vi "Read Error Logger's Enqueuer.vi"(8 "error in (no error)":errorcluster, 11 "TCP_Listener in":refnum<class "TCP_Listener.lvclass">) -> (0 "error out":errorcluster, 2 "Actor Framework:Message Enqueuer":refnum<class "Message Enqueuer.lvclass">, 3 "TCP_Listener out":refnum<class "TCP_Listener.lvclass">)   [LabVIEW 2023, in "TCP_Listener.lvlib" / "TCP_Listener.lvclass"]
uses:
  TCP_Listener.lvclass
  TCP_Listener.lvclass/TCP_Listener.ctl
  <vilib>/ActorFramework/Message Enqueuer/Message Enqueuer.lvclass
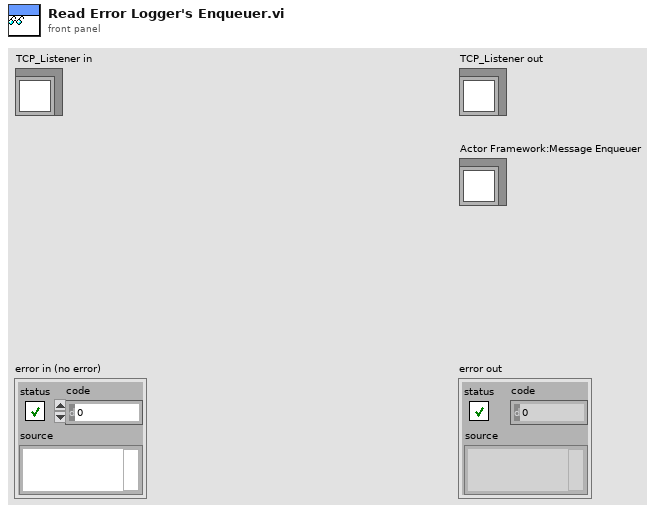
[diagram p1: front panel]
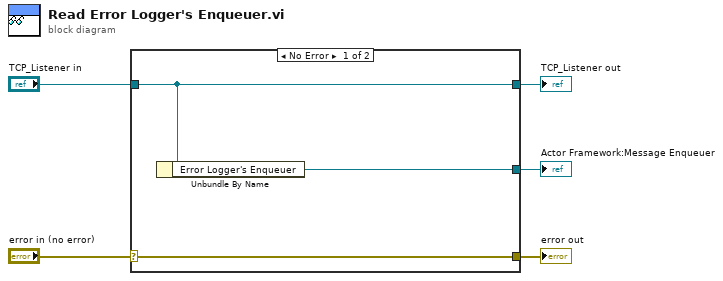
[diagram p0: block diagram]
diagram:
  n1 = case shown="No Error" "error in (no error)" {
    selector: "error in (no error)" -> [w8 w9]
    tunnel: [w8 w9] -> w4
    tunnel: [w7 w10] -> w2
    tunnel: "TCP_Listener in" -> [w7 w10]
    tunnel: [w6 _] -> w1
    frame No Error {
      n2 = Unbundle By Name(w7) -> ("Error Logger's Enqueuer"=w6:refnum<class "Message Enqueuer.lvclass">)
    }
    frame Error {
    }
  }
  "error out" <- w4
  "TCP_Listener out" <- w2
  "Actor Framework:Message Enqueuer" <- w1
